vi "Memory.Constants.vi"   [LabVIEW 2016, in "Memory Manager.lvlib"]
uses:
  Memory Manager.lvlib
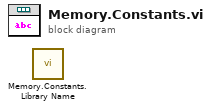
[diagram p0: block diagram]
diagram:
  n1 = call "Memory.Constants.Library Name.vi"() -> ()  [unwired: 11 in, 1 out]
